vi "parseStatus.vi"(8 "error in (no error)":errorcluster, 10 "commandResponse":string, 11 "CoolerSerialCommand in":refnum<class "CoolerSerialCommand.lvclass">) -> (0 "error out":errorcluster, 1 "AS":T2, 2 "PS":T3, 3 "CoolerSerialCommand out":refnum<class "CoolerSerialCommand.lvclass">, 4 "WS":T1, 5 "CS":T4)   [LabVIEW 2016, in "CoolerSerialCommand.lvclass"]
uses:
  CoolerSerialCommand.lvclass
  typedefs/ControlStatusMode.ctl
  typedefs/PumpStatusFlag.ctl
  typedefs/AlarmStatusFlag.ctl
  typedefs/WarningStatusFlag.ctl
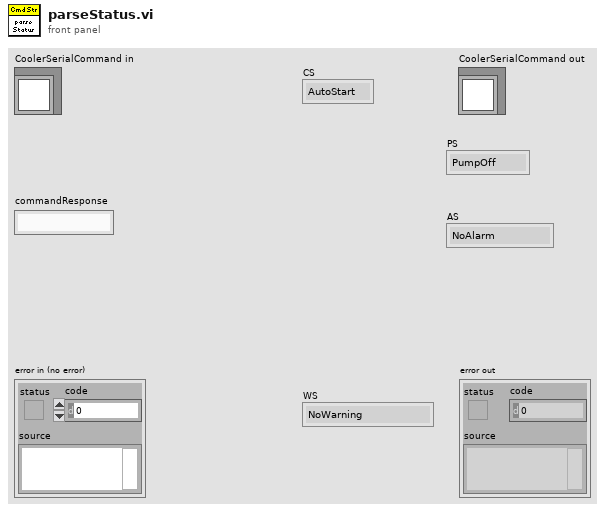
[diagram p1: front panel]
types:
  T1 = typedef "WarningStatusFlag.ctl" = enum16{"NoWarning", "WarningPresent"}
  T2 = typedef "AlarmStatusFlag.ctl" = enum16{"NoAlarm", "AlarmPresent"}
  T3 = typedef "PumpStatusFlag.ctl" = enum16{"PumpOff", "PumpOn"}
  T4 = typedef "ControlStatusMode.ctl" = enum16{"AutoStart", "Standby", "Run", "Safety", "Test"}
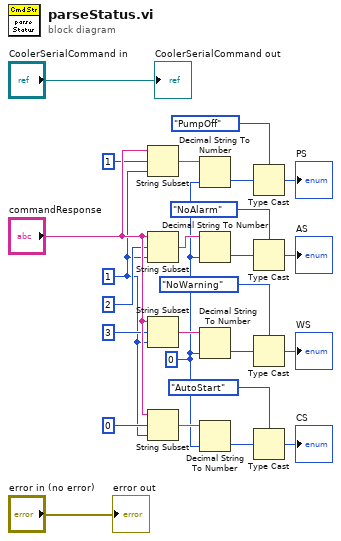
[diagram p0: block diagram]
diagram:
  w9 = u16 0 ("offset (0)")
  w18 = 1 ("length (rest)")
  n1 = String Subset(string="commandResponse", offset (0)=1, length (rest)=w18) -> (substring=w16:string)
  n2 = String Subset(string="commandResponse", offset (0)=2, length (rest)=w18) -> (substring=w15:string)
  n3 = String Subset(string="commandResponse", offset (0)=3, length (rest)=w18) -> (substring=w14:string)
  n4 = String Subset(string="commandResponse", offset (0)=0, length (rest)=w18) -> (substring=w17:string)
  n5 = Decimal String To Number(string=w16, default (0L)=w9) -> (number=w12:u16)  [unwired: 1 in, 1 out]
  n6 = Decimal String To Number(string=w15, default (0L)=w9) -> (number=w11:u16)  [unwired: 1 in, 1 out]
  n7 = Decimal String To Number(string=w14, default (0L)=w9) -> (number=w10:u16)  [unwired: 1 in, 1 out]
  n8 = Decimal String To Number(string=w17, default (0L)=w9) -> (number=w13:u16)  [unwired: 1 in, 1 out]
  n9 = Type Cast(type=PumpStatusFlag."PumpOff" ("PS"), x=w12) -> (*(type *) &x=→"PS":T3)
  n10 = Type Cast(type=AlarmStatusFlag."NoAlarm" ("AS"), x=w11) -> (*(type *) &x=→"AS":T2)
  n11 = Type Cast(type=WarningStatusFlag."NoWarning" ("WS"), x=w10) -> (*(type *) &x=→"WS":T1)
  n12 = Type Cast(type=ControlStatusMode."AutoStart" ("CS"), x=w13) -> (*(type *) &x=→"CS":T4)
  "error out" <- "error in (no error)"
  "CoolerSerialCommand out" <- "CoolerSerialCommand in"
